vi "nPoint_id_slew.vi"() -> ()   [LabVIEW 2017]
uses:
  <vilib>/rvi/Emulation/niFpgaGetClockAttributes.vi
  <vilib>/rvi/Emulation/niFpgaSctlEmulationGetInTimedLoop.vi
  <vilib>/rvi/Emulation/niFpgaEmulationReportErrorSimple.vi
  <vilib>/rvi/eio/common/nirviEmuTemplateMethod_errors.vi
  <vilib>/rvi/interface/RandomDataEmulation/niFpgaRandomDataHandleErrors.vi
  <vilib>/rvi/Emulation/niFpgaCriticalErrorInLSC.vi
  <vilib>/eio/EIONode/EIONode.xnode
  <vilib>/rvi/DataTransferAndStorage/Container/XNode/niFpgaContainer.xnode
  <vilib>/rvi/interface/RandomDataEmulation/nirviRandomDataFpgaReadWriteTemplate.vi
panel:
  in  "yref_k":sgl
  out "YK TO":bool
  out "Unstable Traj":bool
  out "Loop Done":bool
  in  "Abort":bool=TRUE
  in  "ymax":sgl=4.0 format="%#_13g"
  in  "TsTicks":i16
  out "Loop Ticks (benchmark)":i16
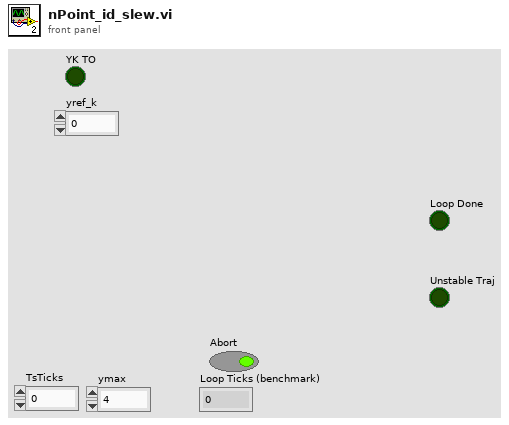
[diagram p1: front panel]
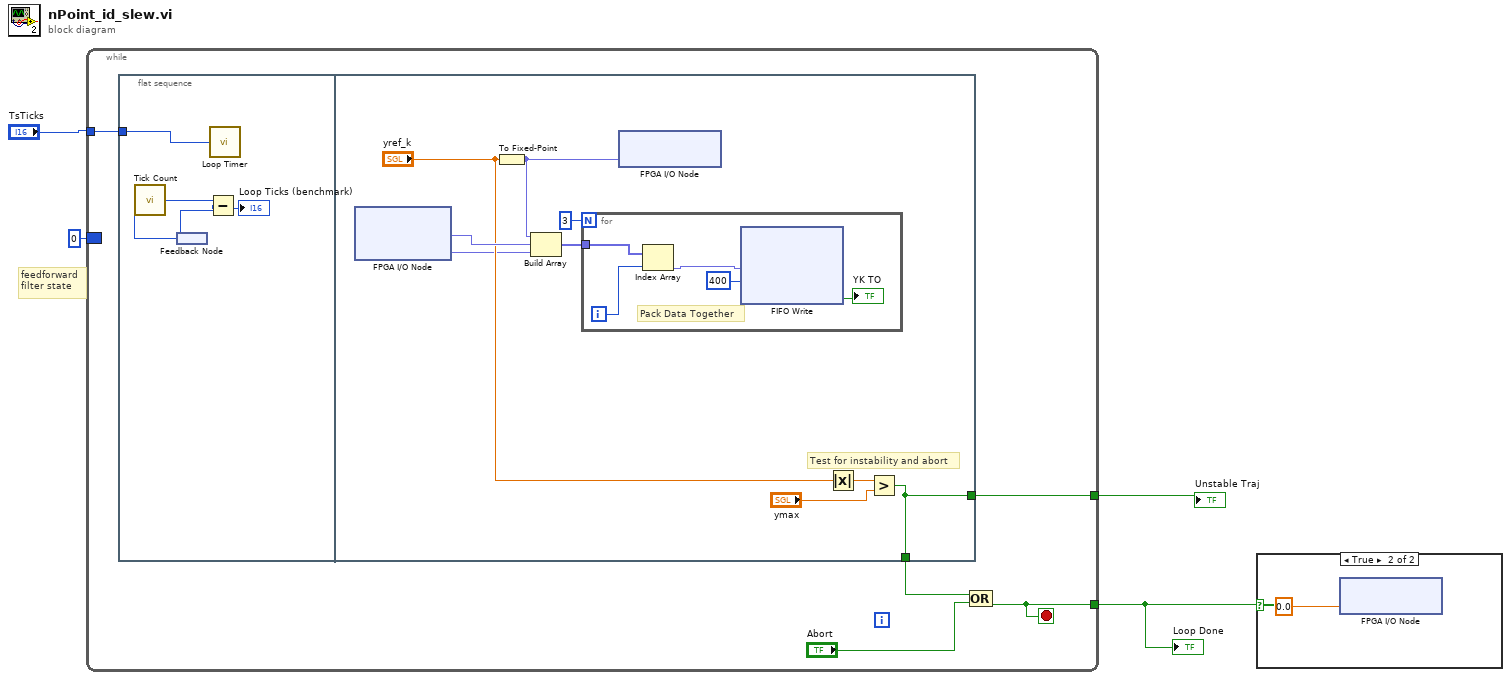
[diagram p0: block diagram]
diagram:
  # "feedforward\nfilter state"
  n1 = while {
    border: i16 0 -> [_]
    tunnel: "TsTicks" -> [w9]
    tunnel: [w6] -> w1
    tunnel: [w8] -> w3
    stop <- w6 stop-if-true
    n2 = flat-sequence {
      tunnel: w9 -> [w10]
      tunnel: [w19] -> w7
      tunnel: [w19] -> w8
      frame #0 {
        n3 = call "Tick Count"() -> ("Tick Count(Ticks)"=w11:u32)
        n4 = feedback #1() -> (w12:u32)
        n5 = feedback-in #1(w11) -> ()
        n6 = Subtract(x=w11, y=w12) -> (x-y=→"Loop Ticks (benchmark)":u32)
        n7 = call "Loop Timer"("Count(Ticks)"=w10) -> ()  [unwired: 1 out]
      }
      frame #1 {
        # "Test for instability and abort"
        n8 = xnode "FPGA I/O Node"() -> ("Mod2/AI0"=w17:fxp<+/-,24,5>, "Mod2/AI1"=w14:fxp<+/-,24,5>)  [unwired: 2 in, 2 out]
        n9 = To Fixed-Point(number="yref_k") -> (fixed-point=w18:fxp<+/-,32,6>)  [unwired: 1 in]
        n10 = Build Array(w18, w17, w14) -> (w20:fxp<+/-,32,6>[])
        n11 = for {
          N: 3 -> [_]
          tunnel: w20 -> [w25]
          i -> [w26]
          # "Pack Data Together"
          n12 = Index Array(array=w25, index=w26) -> (element=w23:fxp<+/-,32,6>)
          n13 = xnode ("FIFO Write")("Element"=w23, "Timeout"=i16 400) -> ("Timed Out?"=→"YK TO":bool)  [unwired: 1 in, 1 out]
        }
        n14 = xnode "FPGA I/O Node"("Mod1/AO0"=w18) -> ()  [unwired: 1 in, 1 out]
        n15 = Absolute Value(x="yref_k") -> (abs(x)=w22:sgl)
        n16 = Greater?(x=w22, y="ymax") -> (0:w19:bool)
      }
    }
    n17 = Compound Arithmetic op=OR(w7, "Abort") -> (w6:bool)
  }
  "Loop Done" <- w1
  "Unstable Traj" <- w3
  n18 = case shown="True" w1 {
    frame False {
    }
    frame True {
      n19 = xnode "FPGA I/O Node"("Mod1/AO0"=sgl 0.0) -> ()  [unwired: 1 in, 1 out]
    }
  }
